vi "Master on Desktop — копия.vi"() -> ()   [LabVIEW 2021]
doc: "Demonstrates how to use Modbus functions to create a master communicating with a Modbus slave. It shows an interactive UI to allow users manually read and write the coils on the slave using TCP connection. Users can also change the timeout for reading operation if the network state is not good."
uses:
  subvis/Modbus API/Modbus API.lvclass/Modbus API.ctl
  subvis/Transmission Data Unit (ADU)/Transmission Data Unit/Transmission Data Unit.lvclass/Transmission Data Unit.ctl
  master/Data Access/Read Timeout/Set Read Timeout.vi
  subvis/Modbus API/Read Transmission Data Unit.vi
  subvis/Modbus API/Write Transmission Data Unit.vi
  subvis/Transmission Data Unit (ADU)/Transmission Data Unit/Data Access/timeouts/Write read operation timeout.vi
  master/Modbus Master.lvclass
  D:/my_projects/projects/Algorithms/Labview/21/Modbus_v2/subvis/Modbus API/Modbus API.lvclass
  master/Create Master Instance (Serial).vi
  subvis/Transmission Data Unit (ADU)/Transmission Data Unit/Transmission Data Unit.lvclass
panel:
  out "register values":u16[](array[numeric])
  in  "Set Read Timeout":bool
  in  "Read Timeout (ms)":i32=5000
  in  "Read Count":u16=10
  in  "Stop":bool
  in  "Read":bool
  out "Coil Values Read":bool[](array[boolean])
  in  "Write":bool
  in  "Coil Values to Write":u16[](array[numeric])
  # "Overview: Demonstrates the use of the Modbus Master VIs to create a Modbus master and use the Modbus master to read and write coil values on a Modbus slave.\nRequirements: LabVIEW Datalogging and Supervisory Control Module\nInstructions:\n1. Ensure Slave On Desktop.vi is already running.\n2. Run the VI.\n3. Click Stop to stop the VI."
  # "Write Operation"
  # "Read Operation"
  # "Set Timeout For Read Operation"
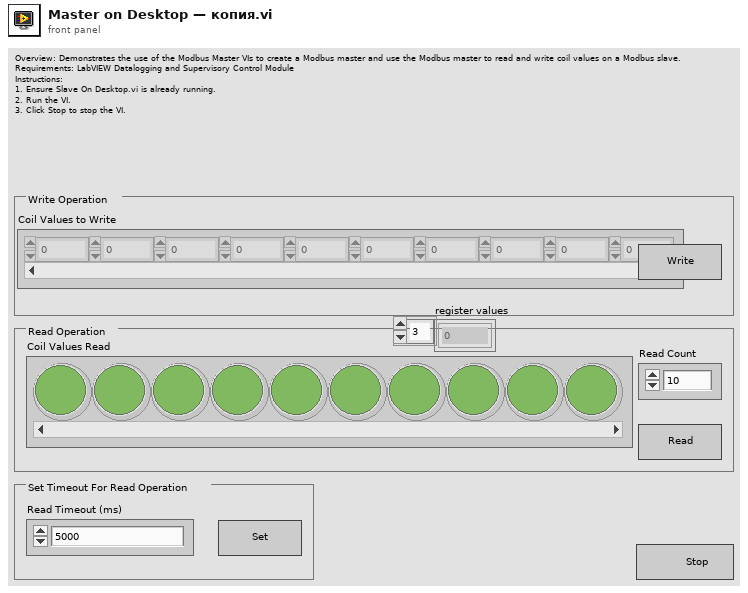
[diagram p1: front panel]
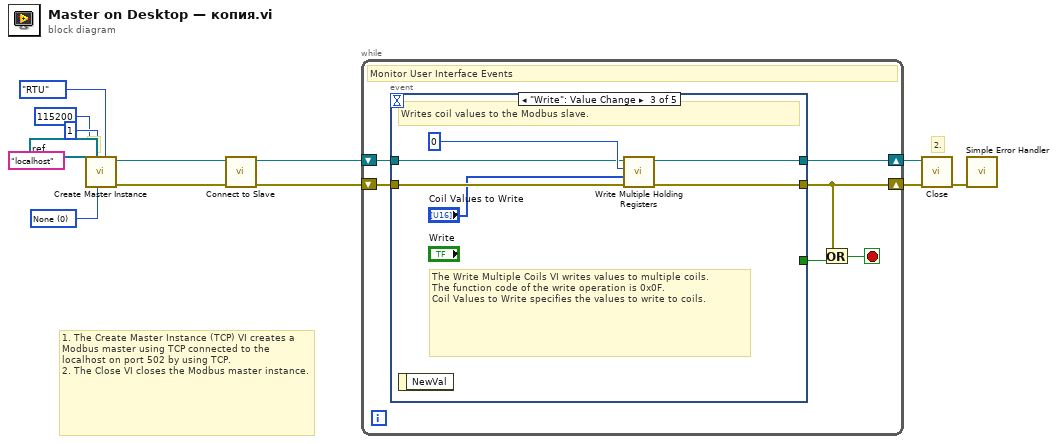
[diagram p0: block diagram]
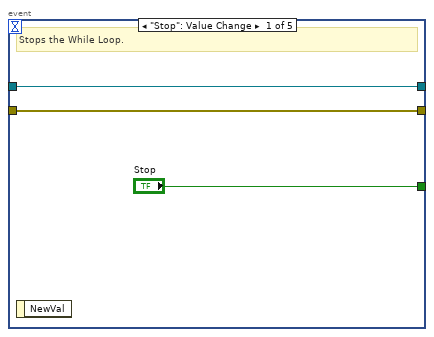
[diagram p2: hidden frame]
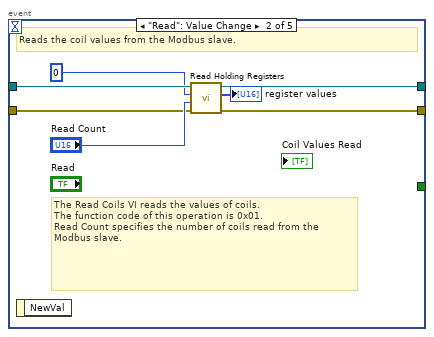
[diagram p3: hidden frame]
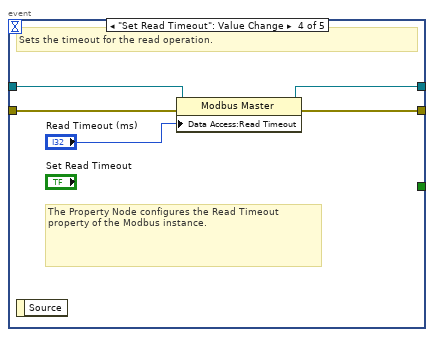
[diagram p4: hidden frame]
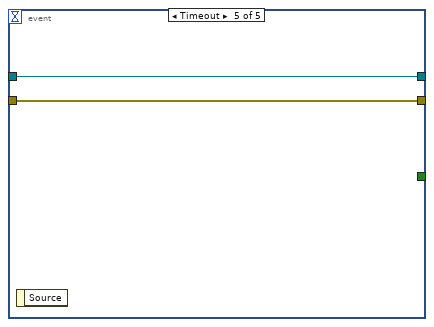
[diagram p5: hidden frame]
diagram:
  w2 = u16 0 items=["None", "Odd", "Even"] ("parity (Even)")
  (unwired) "localhost" ("address")
  # "2."
  # "1."
  # "1. The Create Master Instance (TCP) VI creates a Modbus master using TCP connected to the localhost on port 502 by using TCP.\n2. The Close VI closes the Modbus master instance."
  n1 = call-poly "Create Master Instance.vi"("serial type"=enum16{"RTU", "ASCII"}."RTU", "parity (Even)"=w2, "unit ID"=u8 1, "baud rate (9600)"=u32 115200, "VISA resource name"=refnum<visa-resource-name> "COM18") -> ("error out"=w8:errorcluster, "serial master instance"=w6:refnum<class "Modbus Master.lvclass">)  [unwired: 5 in]
  n2 = call-dynamic "Connect to Slave.vi"("error in (no error)"=w8, "Modbus master in"=w6) -> ("error out"=w7:errorcluster, "Modbus master out"=w9:refnum<class "Modbus Master.lvclass">)  [unwired: 8 in]
  n3 = while {
    shift-right: [w17] -> w11
    shift-left: w9 -> [w18]
    shift-right: [w15] -> w12
    shift-left: w7 -> [w16]
    stop <- w13 stop-if-true
    # "Monitor User Interface Events"
    n4 = event shown="[2] \"Write\": Value Change" {
      selector: _ -> [_ _ _ _ _]
      dyn-events: _ -> [_ _ _ _ _]
      timeout: _ -> [_ _ _ _ _]
      tunnel: ["Stop" _ _ _ _] -> w14
      tunnel: w18 -> [w20 w28 w33 w39 w41]
      tunnel: [w20 w27 w32 w37 w41] -> w17
      tunnel: w16 -> [w21 w24 w31 w38 w40]
      tunnel: [w21 w23 w30 w36 w40] -> w15
      event "Stop": Value Change {
        # "Stops the While Loop."
        n5 = event-data() -> ()  [unwired: 1 in, 1 out]
      }
      event "Read": Value Change {
        # "The Read Coils VI reads the values of coils.\nThe function code of this operation is 0x01.\nRead Count specifies the number of coils read from the Modbus slave."
        # "Reads the coil values from the Modbus slave."
        n6 = event-data() -> ()  [unwired: 1 in, 1 out]
        n7 = call-dynamic "Read Holding Registers.vi"("error in (no error)"=w24, "number of holding registers"="Read Count", "starting address"=u16 0, "Modbus master in"=w28) -> ("error out"=w23:errorcluster, "register values"=→"register values":u16[], "Modbus master out"=w27:refnum<class "Modbus Master.lvclass">)  [unwired: 5 in]
      }
      event "Write": Value Change {
        # "The Write Multiple Coils VI writes values to multiple coils.\nThe function code of the write operation is 0x0F.\nCoil Values to Write specifies the values to write to coils."
        # "Writes coil values to the Modbus slave."
        n8 = event-data() -> ()  [unwired: 1 in, 1 out]
        n9 = call-dynamic "Write Multiple Holding Registers.vi"("error in (no error)"=w31, "holding register values"="Coil Values to Write", "starting address"=u16 0, "Modbus master in"=w33) -> ("error out"=w30:errorcluster, "Modbus master out"=w32:refnum<class "Modbus Master.lvclass">)  [unwired: 6 in]
      }
      event "Set Read Timeout": Value Change {
        # "The Property Node configures the Read Timeout property of the Modbus instance."
        # "Sets the timeout for the read operation."
        n10 = event-data() -> ()  [unwired: 1 in, 1 out]
        n11 = property class="Modbus Master"(reference=w39, error in=w38, "Data Access:Read Timeout"="Read Timeout (ms)") -> (reference out=w37:refnum<class "Modbus Master.lvclass">, error out=w36:errorcluster)
      }
      event Timeout {
        n12 = event-data() -> ()  [unwired: 1 in, 1 out]
      }
    }
    n13 = Or(x=w15, y=w14) -> (x .or. y?=w13:bool)
  }
  n14 = call-dynamic "Close.vi"("error in (no error)"=w12, "Modbus master in"=w11) -> ("error out"=w10:errorcluster)  [unwired: 9 in]
  n15 = call <vilib>:"Simple Error Handler.vi"("error in (no error)"=w10) -> ()  [unwired: 4 in, 5 out]
